vi "Unicode String Probe.vi"(11 "String":string) -> (2 "Value String":string, 3 "Boolean":bool)   [LabVIEW 2020]
uses:
  Unicode/Controls/String Encoding.ctl
  Unicode/Strip BOM.vi
  Unicode/Detect String Encoding.vi/f4e2713d-ca87-487a-b901-d606fc3002c3.vi
  Private/Conversion/Text to UTF-8.vi
  Private/Conversion/Polymorphic VIs/Text to UTF-8 (LabVIEW String).vi
  Private/Conversion/Encoded UTF-8 String to Encoded UTF-16LE String.vi
  Unicode/SubVIs/UTF-16 Byte Swap.vi
  Private/Conversion/UTF-8 to Text.vi
  Private/Conversion/Polymorphic VIs/UTF-8 to Text (LabVIEW String).vi
  Private/Conversion/Encoded UTF-16LE String to Encoded UTF-8 String.vi
  Unicode/SubVIs/Byte Order Marks.vi
  Unicode/Detect BOM.vi
  Private/Library/gu_is_text_utf16.vi
  Private/Library/gu_is_text_utf8.vi
  G-Unicode.lvlib
panel:
  out "Detected Encoding":T1=enum."Unknown"
  out "Unicode":string
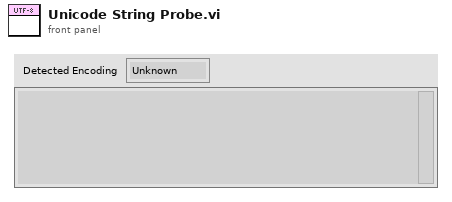
[diagram p1: front panel]
types:
  T1 = typedef "G-Unicode.lvlib/String Encoding.ctl" = enum16{"ANSI", "UTF-8", "UTF-16LE", "UTF-16BE", "Unknown"}
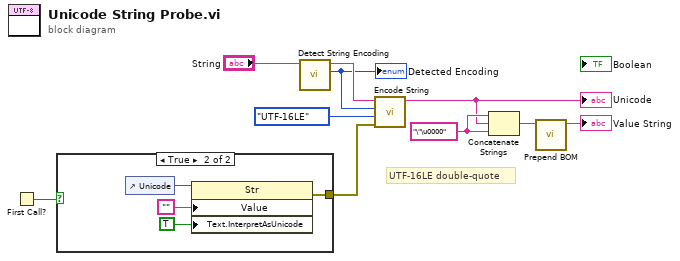
[diagram p0: block diagram]
diagram:
  w7 = "\"\u0000" ("string")
  # "UTF-16LE double-quote"
  n1 = First Call?() -> (First Call?: T/F=w1:bool)
  n2 = case shown="True" w1 {
    tunnel: [_ w14] -> w9
    frame False {
    }
    frame True {
      n3 = control-ref of="Unicode"() -> (w11:refnum<vi>)
      n4 = property on="Property Node" class="Str"(reference=w11, "Value"="", "Text.InterpretAsUnicode"=TRUE ("Force Unicode Text")) -> (error out=w14:errorcluster)  [unwired: 1 in, 1 out]
    }
  }
  n5 = call "Detect String Encoding.vi"("String"="String") -> ("Encoding"=w2:T1, "String out"=w3:string)  [unwired: 8 in, 1 out]
  "Detected Encoding" <- w2
  n6 = call "Encode String.vi"("error in"=w9, "Output Encoding (UTF-16LE)"=String_Encoding."UTF-16LE" ("Output Encoding (UTF-8)"), "Input Encoding (ANSI)"=w2, "String in"=w3) -> ("String out"=w6:string)  [unwired: 6 in, 1 out]
  "Unicode" <- w6
  n7 = Concatenate Strings(w7, w6, w7) -> (w5:string)
  n8 = call "Prepend BOM.vi"("String"=w5) -> ("String with BOM"=→"Value String":string)  [unwired: 9 in, 1 out]
